vi "Name.vi"(8 "error in (no error)":errorcluster, 11 "Output Actor Hardware in":refnum<class "Output Actor Hardware.lvclass">) -> (0 "error out":errorcluster, 2 "Name":string, 3 "Output Actor Hardware out":refnum<class "Output Actor Hardware.lvclass">)   [LabVIEW 2015, in "Output Actor Hardware.lvclass"]
uses:
  Output Actor Hardware.lvclass
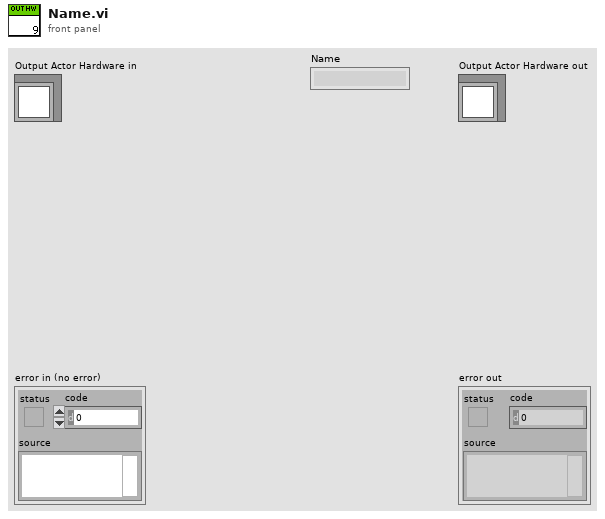
[diagram p1: front panel]
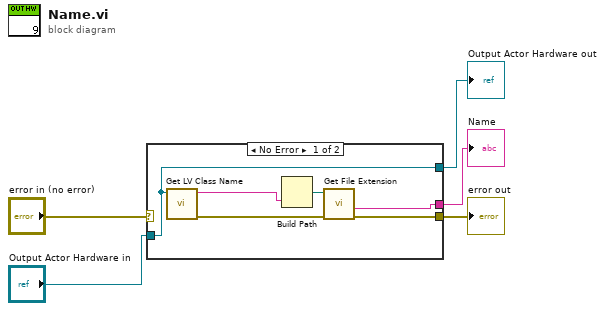
[diagram p0: block diagram]
diagram:
  n1 = case shown="No Error" "error in (no error)" {
    selector: "error in (no error)" -> [_ w13]
    tunnel: [w7 w13] -> w4
    tunnel: [w11 w12] -> w2
    tunnel: "Output Actor Hardware in" -> [w11 w12]
    tunnel: [w6 _] -> w1
    frame No Error {
      n2 = call <vilib>:"Get LV Class Name.vi"("object"=w11) -> ("error out"=w8:errorcluster, "class name"=w10:string)  [unwired: 9 in]
      n3 = Build Path(name or relative path=w10) -> (appended path=w9:path)  [unwired: 1 in]
      n4 = call <vilib>:"Get File Extension.vi"("error in (no error)"=w8, "file"=w9) -> ("error out"=w7:errorcluster, "filename without extension"=w6:string)  [unwired: 5 in, 3 out]
    }
    frame Error {
    }
  }
  "error out" <- w4
  "Output Actor Hardware out" <- w2
  "Name" <- w1
